vi "rs3 get option range.vi"(8 "error in (no error)":errorcluster, 10 "RS Option":u16(ring) items=["    RS2_OPTION_BACKLIGHT_COMPENSATION                     , /**< Enable / disable color backlight compensation*/", "    RS2_OPTION_BRIGHTNESS                                 , /**< Color image brightness*/", "    RS2_OPTION_CONTRAST                                   , /**< Color image contrast*/", "    RS2_OPTION_EXPOSURE                                   , /**< Controls exposure time of color camera. Setting any value will disable auto exposure*/", "    RS2_OPTION_GAIN                                       , /**< Color image gain*/", "    RS2_OPTION_GAMMA                                      , /**< Color image gamma setting*/", "    RS2_OPTION_HUE                                        , /**< Color image hue*/", "    RS2_OPTION_SATURATION                                 , /**< Color image saturation setting*/", "    RS2_OPTION_SHARPNESS                                  , /**< Color image sharpness setting*/", "    RS2_OPTION_WHITE_BALANCE                              , /**< Controls white balance of color image. Setting any value will disable auto white balance*/", "    RS2_OPTION_ENABLE_AUTO_EXPOSURE                       , /**< Enable / disable color image auto-exposure*/", "    RS2_OPTION_ENABLE_AUTO_WHITE_BALANCE                  , /**< Enable / disable color image auto-white-balance*/", "    RS2_OPTION_VISUAL_PRESET                              , /**< Provide access to several recommend sets of option presets for the depth camera */", "    RS2_OPTION_LASER_POWER                                , /**< Power of the F200 / SR300 projector, with 0 meaning projector off*/", "    RS2_OPTION_ACCURACY                                   , /**< Set the number of patterns projected per frame. The higher the accuracy value the more patterns projected. Increasing the number of patterns help to achieve better accuracy. Note that this c", "    RS2_OPTION_MOTION_RANGE                               , /**< Motion vs. Range trade-off, with lower values allowing for better motion sensitivity and higher values allowing for better depth range*/", "    RS2_OPTION_FILTER_OPTION                              , /**< Set the filter to apply to each depth frame. Each one of the filter is optimized per the application requirements*/", "    RS2_OPTION_CONFIDENCE_THRESHOLD                       , /**< The confidence level threshold used by the Depth algorithm pipe to set whether a pixel will get a valid range or will be marked with invalid range*/", "    RS2_OPTION_EMITTER_ENABLED                            , /**< Laser Emitter enabled */", "    RS2_OPTION_FRAMES_QUEUE_SIZE                          , /**< Number of frames the user is allowed to keep per stream. Trying to hold-on to more frames will cause frame-drops.*/", "    RS2_OPTION_TOTAL_FRAME_DROPS                          , /**< Total number of detected frame drops from all streams */", "    RS2_OPTION_AUTO_EXPOSURE_MODE                         , /**< Auto-Exposure modes: Static, Anti-Flicker and Hybrid */", "    RS2_OPTION_POWER_LINE_FREQUENCY                       , /**< Power Line Frequency control for anti-flickering Off/50Hz/60Hz/Auto */", "    RS2_OPTION_ASIC_TEMPERATURE                           , /**< Current Asic Temperature */", "    RS2_OPTION_ERROR_POLLING_ENABLED                      , /**< disable error handling */", "    RS2_OPTION_PROJECTOR_TEMPERATURE                      , /**< Current Projector Temperature */", "    RS2_OPTION_OUTPUT_TRIGGER_ENABLED                     , /**< Enable / disable trigger to be outputed from the camera to any external device on every depth frame */", "    RS2_OPTION_MOTION_MODULE_TEMPERATURE                  , /**< Current Motion-Module Temperature */", "    RS2_OPTION_DEPTH_UNITS                                , /**< Number of meters represented by a single depth unit */", "    RS2_OPTION_ENABLE_MOTION_CORRECTION                   , /**< Enable/Disable automatic correction of the motion data */", "    RS2_OPTION_AUTO_EXPOSURE_PRIORITY                     , /**< Allows sensor to dynamically ajust the frame rate depending on lighting conditions */", "    RS2_OPTION_COLOR_SCHEME                               , /**< Color scheme for data visualization */", "    RS2_OPTION_HISTOGRAM_EQUALIZATION_ENABLED             , /**< Perform histogram equalization post-processing on the depth data */", "    RS2_OPTION_MIN_DISTANCE                               , /**< Minimal distance to the target */", "    RS2_OPTION_MAX_DISTANCE                               , /**< Maximum distance to the target */", "    RS2_OPTION_TEXTURE_SOURCE                             , /**< Texture mapping stream unique ID */", "    RS2_OPTION_FILTER_MAGNITUDE                           , /**< The 2D-filter effect. The specific interpretation is given within the context of the filter */", "    RS2_OPTION_FILTER_SMOOTH_ALPHA                        , /**< 2D-filter parameter controls the weight/radius for smoothing.*/", "    RS2_OPTION_FILTER_SMOOTH_DELTA                        , /**< 2D-filter range/validity threshold*/", "    RS2_OPTION_HOLES_FILL                                 , /**< Enhance depth data post-processing with holes filling where appropriate*/", "    RS2_OPTION_STEREO_BASELINE                            , /**< The distance in mm between the first and the second imagers in stereo-based depth cameras*/", "    RS2_OPTION_AUTO_EXPOSURE_CONVERGE_STEP                , /**< Allows dynamically ajust the converge step value of the target exposure in Auto-Exposure algorithm*/", "    RS2_OPTION_COUNT                                        /**< Number of enumeration values. Not a valid input: intended to be used in for-loops. */"], 11 "Sensor in":u64) -> (0 "error out":errorcluster, 1 "error":u64, 3 "Sensor out":u64, 4 "Default":sgl, 5 "Max":sgl, 6 "Step":sgl, 7 "Min":sgl)   [LabVIEW 2017, in "libRealSense3.lvlib"]
doc: "Retrieves the valid range and default value for the specified sensor option.\n \nInput:\noption the option whose value to set\n \nOutput:\nmin min acceptable\nmax max acceptable\nstep step size\ndefault default value if not set\nerror if non-null, receives any error that occurs during this call, otherwise, errors are ignored"
uses:
  libRealSense3.lvlib
  realsense2.dll
panel:
  # "typedef enum rs2_option\n{\n    RS2_OPTION_BACKLIGHT_COMPENSATION                     , /**< Enable / disable color backlight compensation*/\n    RS2_OPTION_BRIGHTNESS                                 , /**< Color image brightness*/\n    RS2_OPTION_CONTRAST                                   , /**< Color image contrast*/\n    RS2_OPTION_EXPOSURE                                   , /**< Controls exposure time of color camera. Setting any value will disable auto exposure*/\n    RS2_OPTION_GAIN                                       , /**< Color image gain*/\n    RS2_OPTION_GAMMA                                      , /**< Color image gamma setting*/\n    RS2_OPTION_HUE                                        , /**< Color image hue*/\n    RS2_OPTION_SATURATION                                 , /**< Color image saturation setting*/\n    RS2_OPTION_SHARPNESS                                  , /**< Color image sharpness setting*/\n    RS2_OPTION_WHITE_BALANCE                              , /**< Controls white balance of color image. Setting any value will disable auto white balance*/\n    RS2_OPTION_ENABLE_AUTO_EXPOSURE                       , /**< Enable / disable color image auto-exposure*/\n    RS2_OPTION_ENABLE_AUTO_WHITE_BALANCE                  , /**< Enable / disable color image auto-white-balance*/\n    RS2_OPTION_VISUAL_PRESET                              , /**< Provide access to several recommend sets of option presets for the depth camera */\n    RS2_OPTION_LASER_POWER                                , /**< Power of the F200 / SR300 projector, with 0 meaning projector off*/\n    RS2_OPTION_ACCURACY                                   , /**< Set the number of patterns projected per frame. The higher the accuracy value the more patterns projected. Increasing the number of patterns help to achieve better accuracy. Note that this control is affecting the Depth FPS */\n    RS2_OPTION_MOTION_RANGE                               , /**< Motion vs. Range trade-off, with lower values allowing for better motion sensitivity and higher values allowing for better depth range*/\n    RS2_OPTION_FILTER_OPTION                              , /**< Set the filter to apply to each depth frame. Each one of the filter is optimized per the application requirements*/\n    RS2_OPTION_CONFIDENCE_THRESHOLD                       , /**< The confidence level threshold used by the Depth algorithm pipe to set whether a pixel will get a valid range or will be marked with invalid range*/\n    RS2_OPTION_EMITTER_ENABLED                            , /**< Laser Emitter enabled */\n    RS2_OPTION_FRAMES_QUEUE_SIZE                          , /**< Number of frames the user is allowed to keep per stream. Trying to hold-on to more frames will cause frame-drops.*/\n    RS2_OPTION_TOTAL_FRAME_DROPS                          , /**< Total number of detected frame drops from all streams */\n    RS2_OPTION_AUTO_EXPOSURE_MODE                         , /**< Auto-Exposure modes: Static, Anti-Flicker and Hybrid */\n    RS2_OPTION_POWER_LINE_FREQUENCY                       , /**< Power Line Frequency control for anti-flickering Off/50Hz/60Hz/Auto */\n    RS2_OPTION_ASIC_TEMPERATURE                           , /**< Current Asic Temperature */\n    RS2_OPTION_ERROR_POLLING_ENABLED                      , /**< disable error handling */\n    RS2_OPTION_PROJECTOR_TEMPERATURE                      , /**< Current Projector Temperature */\n    RS2_OPTION_OUTPUT_TRIGGER_ENABLED                     , /**< Enable / disable trigger to be outputed from the camera to any external device on every depth frame */\n    RS2_OPTION_MOTION_MODULE_TEMPERATURE                  , /**< Current Motion-Module Temperature */\n    RS2_OPTION_DEPTH_UNITS                                , /**< Number of meters represented by a single depth unit */\n    RS2_OPTION_ENABLE_MOTION_CORRECTION                   , /**< Enable/Disable automatic correction of the motion data */\n    RS2_OPTION_AUTO_EXPOSURE_PRIORITY                     , /**< Allows sensor to dynamically ajust the frame rate depending on lighting conditions */\n    RS2_OPTION_COLOR_SCHEME                               , /**< Color scheme for data visualization */\n    RS2_OPTION_HISTOGRAM_EQUALIZATION_ENABLED             , /**< Perform histogram equalization post-processing on the depth data */\n    RS2_OPTION_MIN_DISTANCE                               , /**< Minimal distance to the target */\n    RS2_OPTION_MAX_DISTANCE                               , /**< Maximum distance to the target */\n    RS2_OPTION_TEXTURE_SOURCE                             , /**< Texture mapping stream unique ID */\n    RS2_OPTION_FILTER_MAGNITUDE                           , /**< The 2D-filter effect. The specific interpretation is given within the context of the filter */\n    RS2_OPTION_FILTER_SMOOTH_ALPHA                        , /**< 2D-filter parameter controls the weight/radius for smoothing.*/\n    RS2_OPTION_FILTER_SMOOTH_DELTA                        , /**< 2D-filter range/validity threshold*/\n    RS2_OPTION_HOLES_FILL                                 , /**< Enhance depth data post-processing with holes filling where appropriate*/\n    RS2_OPTION_STEREO_BASELINE                            , /**< The distance in mm between the first and the second imagers in stereo-based depth cameras*/\n    RS2_OPTION_AUTO_EXPOSURE_CONVERGE_STEP                , /**< Allows dynamically ajust the converge step value of the target exposure in Auto-Exposure algorithm*/\n    RS2_OPTION_COUNT                                        /**< Number of enumeration values. Not a valid input: intended to be used in for-loops. */\n} rs2_option;"
  # "RS3 Get Option Range"
  # "(C) 2018 Intel Corp.,  AGJ"
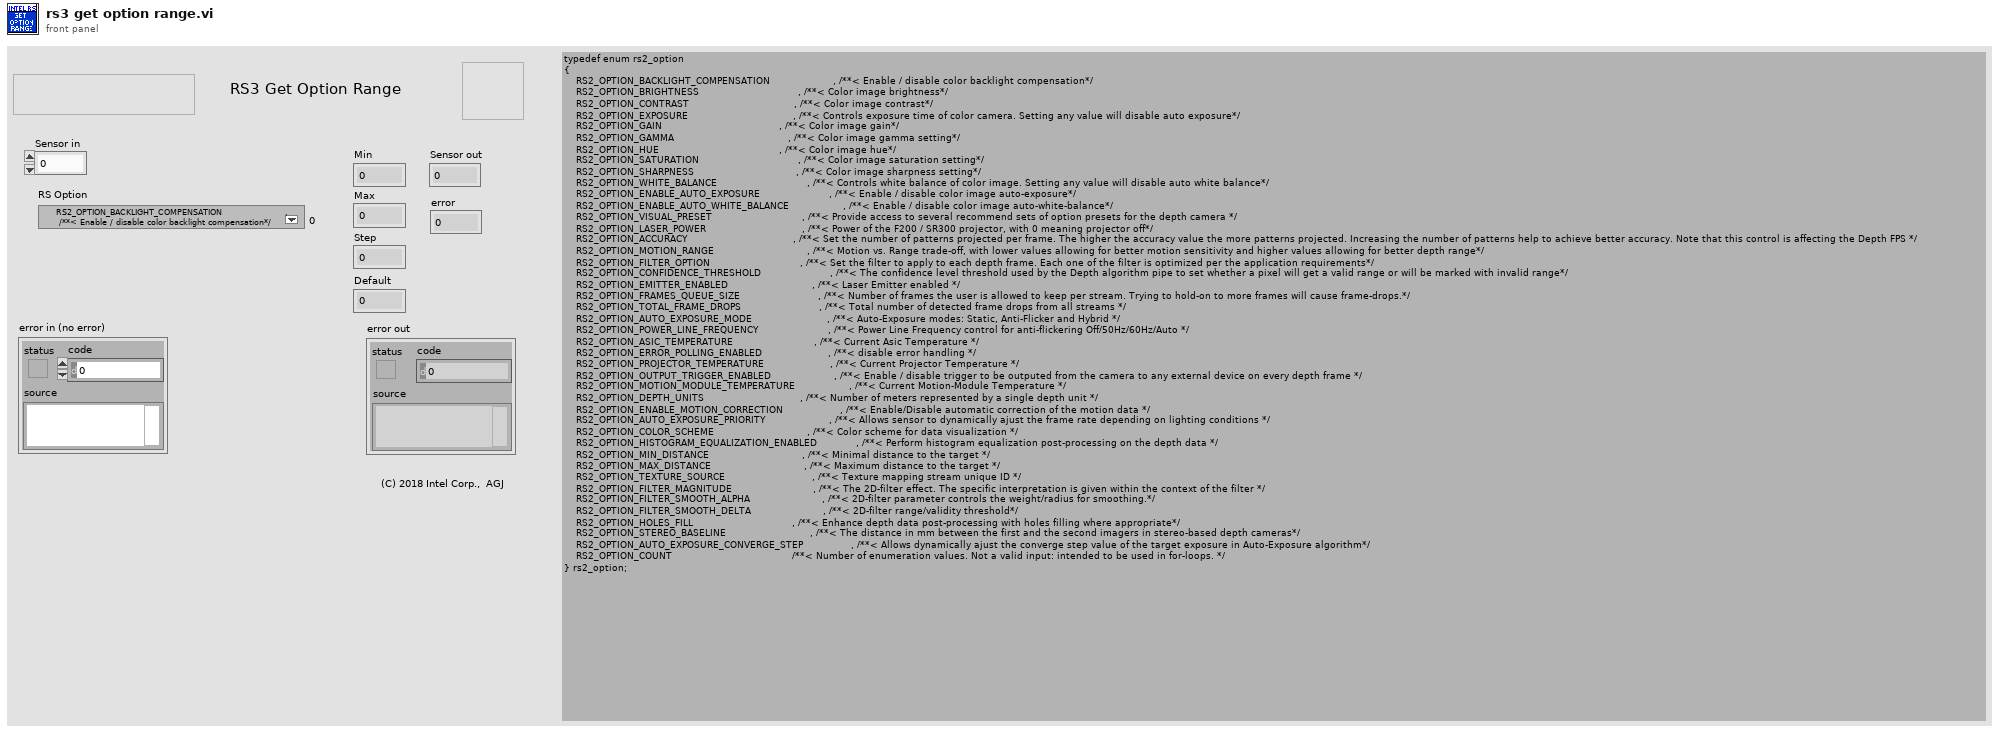
[diagram p1: front panel]
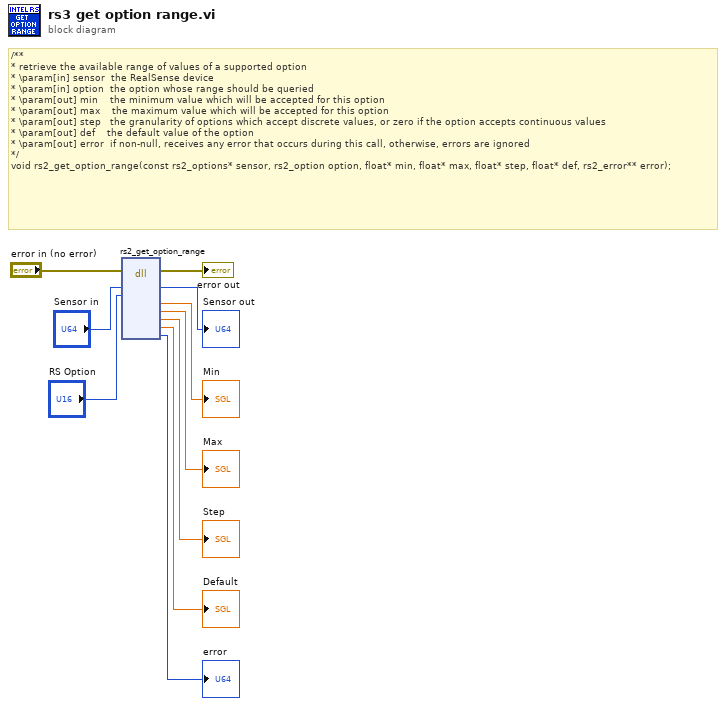
[diagram p0: block diagram]
diagram:
  # "/**\n* retrieve the available range of values of a supported option\n* \\param[in] sensor  the RealSense device\n* \\param[in] option  the option whose range should be queried\n* \\param[out] min    the minimum value which will be accepted for this option\n* \\param[out] max    the maximum value which will be accepted for this option\n* \\param[out] step   the granularity of options which accept discrete values, or zero if the option accepts continuous values\n* \\param[out] def    the default value of the option\n* \\param[out] error  if non-null, receives any error that occurs during this call, otherwise, errors are ignored\n*/\nvoid rs2_get_option_range(const rs2_options* sensor, rs2_option option, float* min, float* max, float* step, float* def, rs2_error** error);"
  n1 = dll-call lib="C:/Users/smartek/Desktop/labview/realsense2.dll" fn="rs2_get_option_range"(error in="error in (no error)", "sensor"="Sensor in", "option"="RS Option") -> (error out=→"error out":errorcluster, "sensor"=→"Sensor out":u64, "Min"=→"Min":sgl, "Max"=→"Max":sgl, "Step"=→"Step":sgl, "Default"=→"Default":sgl, "error"=→"error":u64)  [unwired: 9 in, 1 out]
